vi "VFH-get_all_file_paths.vi"(8 "error in (no error)":errorcluster, 10 "Folder Path":path) -> (0 "error out":errorcluster, 1 "empty?":bool, 2 "All Files in Dir":path[](array[path]))   [LabVIEW 2020, in "VFH-VNA_File_Handler.lvlib"]
uses:
  VFH-VNA_File_Handler.lvlib
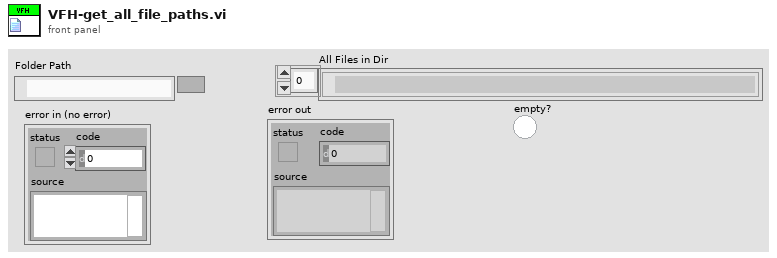
[diagram p1: front panel]
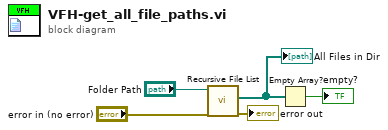
[diagram p0: block diagram]
diagram:
  n1 = call <vilib>:"Recursive File List.vi"("error in (no error)"="error in (no error)", "Folder Path"="Folder Path") -> ("error out"=→"error out":errorcluster, "All Files in Dir"=w2:path[])  [unwired: 5 in, 3 out]
  "All Files in Dir" <- w2
  n2 = Empty Array?(array=w2) -> (empty?=→"empty?":bool)
